vi "CTRE_Phoenix_CANCoder_GetUnitString.vi"(6 "timeoutMs":i32, 8 "error in":errorcluster, 11 "CTRE_CANcoder_DeviceRef":T1) -> (0 "error out":errorcluster, 2 "Unit String":string, 3 "CTRE_CANcoder_DeviceRef":T1)   [LabVIEW 2020]
doc: "Returns the absolute position of the CANcoder."
uses:
  <vilib>/Rock Robotics/WPI/ThirdParty/Phoenix-LabVIEW/CANCoder/Controls/CTRE_Phoenix_CANcoder_DeviceRef.ctl
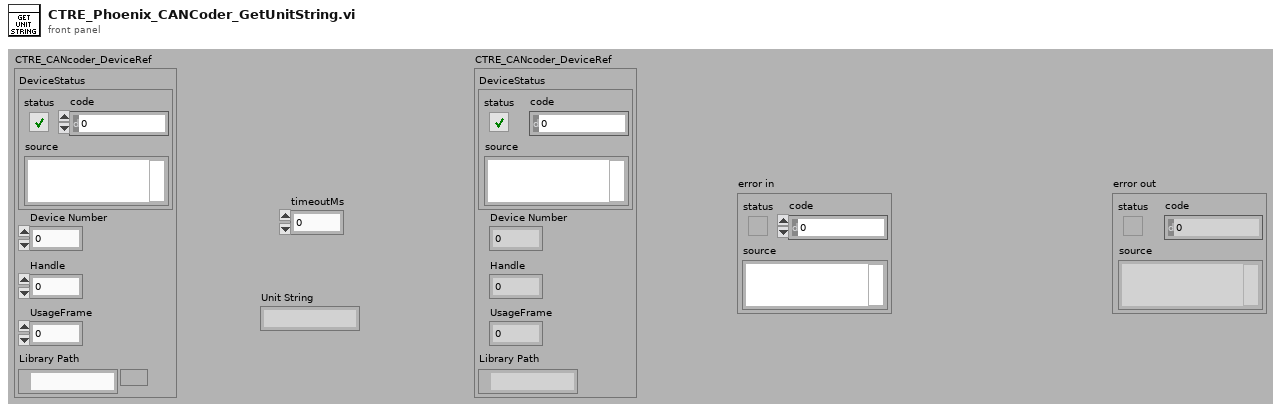
[diagram p1: front panel]
types:
  T1 = typedef "CTRE_Phoenix_CANcoder_DeviceRef.ctl" = cluster{"DeviceStatus":errorcluster, "Device Number":u8, "Handle":u64, "UsageFrame":u32, "Library Path":path}
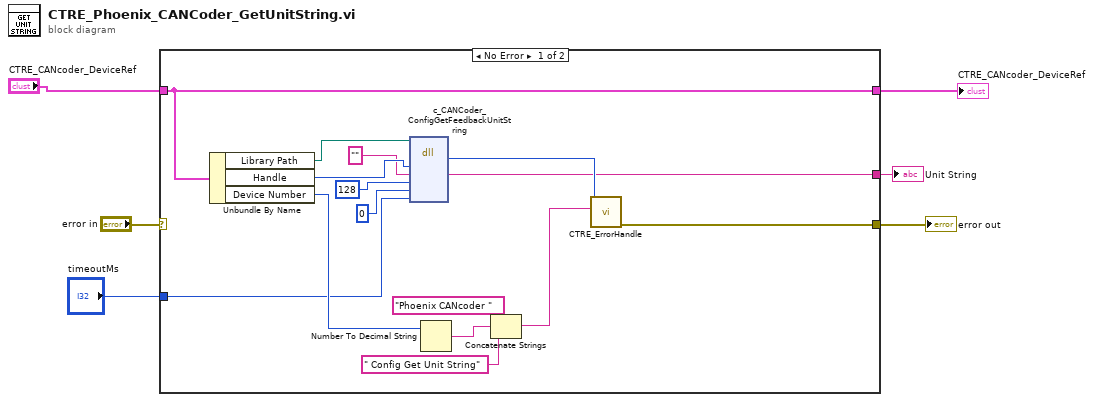
[diagram p0: block diagram]
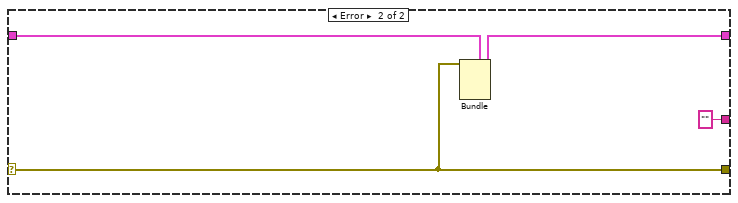
[diagram p2: hidden frame]
diagram:
  n1 = case shown="No Error" "error in" {
    selector: "error in" -> [_ w24]
    tunnel: "CTRE_CANcoder_DeviceRef" -> [w15 w25]
    tunnel: [w21 w24] -> w6
    tunnel: [w15 w23] -> w3
    tunnel: [w11 "" ("unitStringToFill")] -> w2
    tunnel: "timeoutMs" -> [w10 _]
    frame No Error {
      n2 = Unbundle By Name(w15) -> ("Library Path"=w13:path, "Handle"=w12:u64, "Device Number"=w14:u8)
      n3 = dll-call lib="?" fn="c_CANCoder_ConfigGetFeedbackUnitString"(path in=w13, "handle"=w12, "unitStringToFill"="", "toFillByteSz"=128, "numBytesFilled"=0, "timeoutMs"=w10) -> ("return type"=w17:i32, "unitStringToFill"=w11:string)  [unwired: 6 in, 2 out]
      n4 = Number To Decimal String(number=w14) -> (decimal integer string=w19:string)  [unwired: 1 in]
      n5 = Concatenate Strings("Phoenix CANcoder " ("string"), w19, " Config Get Unit String" ("string")) -> (w16:string)
      n6 = call <vilib>:"CTRE_ErrorHandle.vi"("origin"=w16, "code"=w17) -> ("error out"=w21:errorcluster)  [unwired: 9 in]
    }
    frame Error {
      n7 = Bundle(cluster=w25, "DeviceStatus"=w24) -> (w23:T1)  [unwired: 4 in]
    }
  }
  "error out" <- w6
  "CTRE_CANcoder_DeviceRef" <- w3
  "Unit String" <- w2
